vi "RobotRunTest 1 arm.vi"() -> ()   [LabVIEW 2016]
uses:
  EyeRobotDLL.dll
panel:
  in  "Auto Home":bool
  in  "KillControlProcess(for debug only)":bool
  out "ROBOT_KINEMATICS_NO_SOLUTION":bool
  out "ROBOT_KINEMATICS_INSERTION_LENGTH_TOO_SMALL":bool
  out "ROBOT_COMMAND_BEYONG_JOINT_RANGE":bool
  out "ROBOT_COMMAND_TOO_LARGE":bool
  out "ROBOT_COMMUNICATION_ERROR":bool
  out "ROBOT_NOT_RUNNING":bool
  out "ROBOT_HARDWARE_SENSOR_FAULT":bool
  out "ROBOT_HARDWARE_NOT_FOUND_ALL_DRIVES":bool
  out "ROBOT_HARDWARE_NOT_PRESENT":bool
  in  "ToolInsertionOffset":dbl=-54.76
  out "Homing XYZ Stage Done":bool
  out "Homing Tool Done":bool
  out "Homing Arm Done":bool
  out "Actual Tool Insertion Length":dbl
  in  "Tool Withdraw":bool
  in  "Target Tool Withdraw Speed":dbl=0.5
  in  "Target Tool Withdraw Length":dbl=-5.0
  in  "Set Tool Type":bool
  in  "ToolType":i32=6
  in  "Tool Fast Retraction":bool
  in  "Tool Insertion":bool
  in  "Target Tool Insertion Speed":dbl=0.5
  in  "Target Tool Insertion Length":dbl=10.0
  in  "Homing XYZ Stage":bool
  in  "Homing Tool":bool
  in  "Homing Arm":bool
  in  "XYZ Control or Joint Control":bool
  in  "E-STOP button":bool caption="Stop Button"
  in  "Robot Command":T1={"x"=0.0, "y"=0.0, "z"=-10.0, "roll"=0.0, "grasp"=0.0}
  in  "joint command":T2
  in  "Stop Labview Button":bool caption="Stop Button"
  in  "Run Pause":bool
  in  "XYZ Stage Power":bool
  in  "ArmPower":bool
  in  "XYZ Stage Command":cluster{"x":dbl, "y":dbl, "z":dbl}
  out "XYZ Stage Data":cluster{"x":dbl, "y":dbl, "z":dbl}
  out "Robot Data":T1
  out "ActualJointAngles (8 DOF)":T2
  out "RobotConnection Status":bool
  out "ReceiveCount":u64
  out "SendCount":u64
  # "Robot XYZ Command (kinematics included)"
  # "Joint Angle Command (for debug and testing)"
  # "Robot Status"
  # "XYZ Stage Position"
  # "Tool Insertion Commands"
  # "Homing Commands"
  # "Robot Errors"
  # "Tool Configuration Commands"
  # "For debug only, No need to use this button during labview operation, if does, then the low level control will be terminated, and everything will have to be rerestarted including homing"
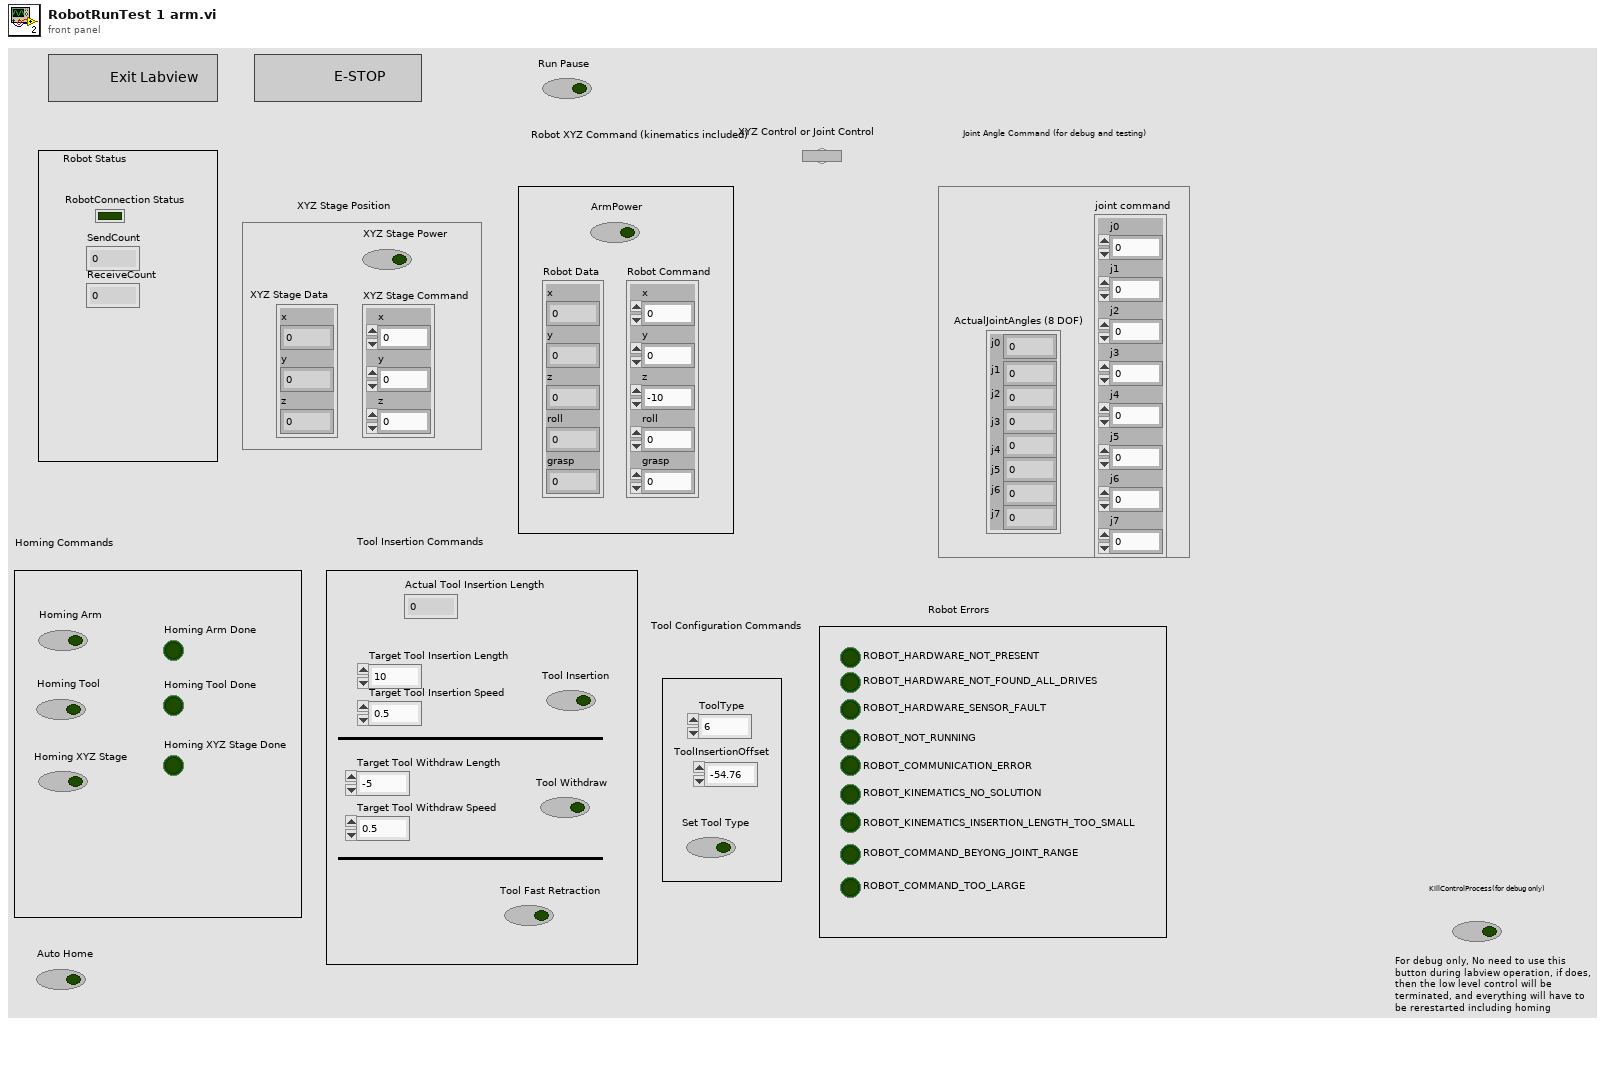
[diagram p1: front panel]
types:
  T1 = cluster{"x":dbl, "y":dbl, "z":dbl, "roll":dbl, "grasp":dbl}
  T2 = cluster{"j0":dbl, "j1":dbl, "j2":dbl, "j3":dbl, "j4":dbl, "j5":dbl, "j6":dbl, "j7":dbl}
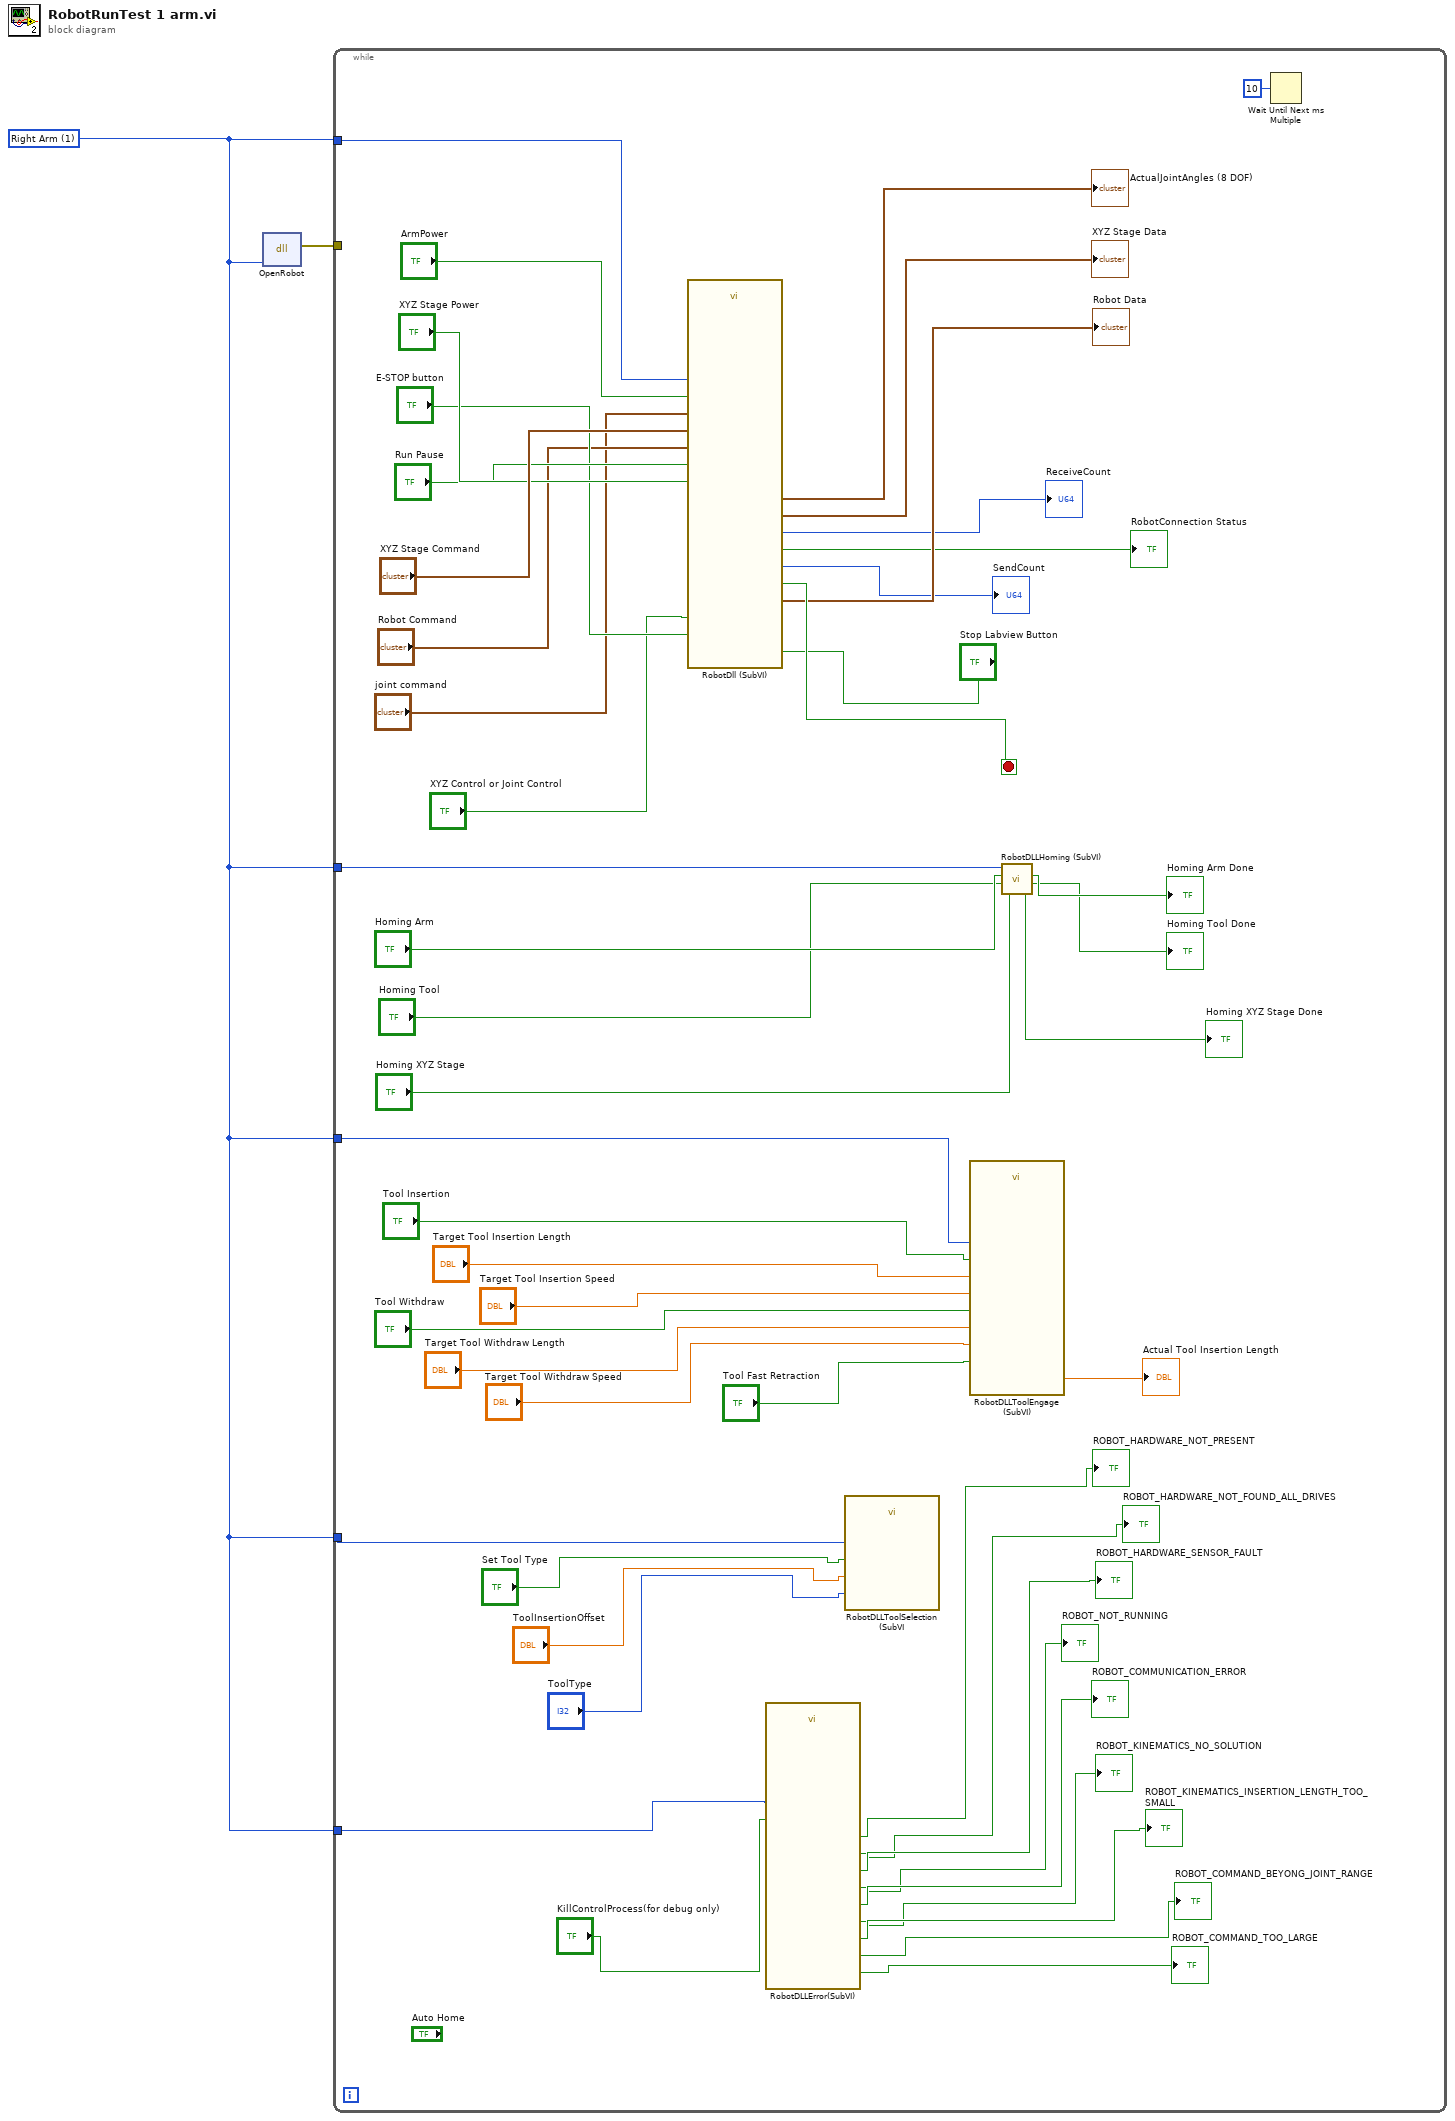
[diagram p0: block diagram]
diagram:
  w1 = u16 1 items=["Left Arm", "Right Arm"] ("Left or Right Arm")
  n1 = dll-call lib="D:/IRISS V2 dev/Host Demo/Functions/EyeRobotDLL.dll" fn="OpenRobot" label="Open"("id"=w1) -> (error out=w2:errorcluster)  [unwired: 5 in, 1 out]
  n2 = while {
    tunnel: w2 -> [_]
    tunnel: w1 -> [w45]
    tunnel: w1 -> [w24]
    tunnel: w1 -> [w33]
    tunnel: w1 -> [w7]
    tunnel: w1 -> [w3]
    stop <- w46 stop-if-true
    n3 = call "RobotDll (SubVI).vi"("rcm xyz command"="XYZ Stage Command", "ArmPower"="ArmPower", "Control Mode"="XYZ Control or Joint Control", "XYZ Stage Power"="XYZ Stage Power", "E-STOP button"="E-STOP button", "robot xyz command"="Robot Command", "ArmID"=w45, "Run"="Run Pause", "Stop Button in"="Stop Labview Button", "joint command"="joint command") -> ("rcm"=→"XYZ Stage Data":cluster{"x":dbl, "y":dbl, "z":dbl}, "Stop Button out"=w46:bool, "Tooltip"=→"Robot Data":T1, "ReceiveCount"=→"ReceiveCount":u64, "ActualJointAngles"=→"ActualJointAngles (8 DOF)":T2, "SendCount"=→"SendCount":u64, "RobotConnection"=→"RobotConnection Status":bool)  [unwired: 3 in]
    n4 = call "RobotDLLError(SubVI).vi"("ArmID"=w3, "KillRobotControlProcess"="KillControlProcess(for debug only)") -> ("ROBOT_COMMAND_BEYONG_JOINT_RANGE"=→"ROBOT_COMMAND_BEYONG_JOINT_RANGE":bool, "ROBOT_KINEMATICS_NO_SOLUTION"=→"ROBOT_KINEMATICS_NO_SOLUTION":bool, "ROBOT_HARDWARE_NOT_PRESENT"=→"ROBOT_HARDWARE_NOT_PRESENT":bool, "ROBOT_HARDWARE_NOT_FOUND_ALL_DRIVES"=→"ROBOT_HARDWARE_NOT_FOUND_ALL_DRIVES":bool, "ROBOT_HARDWARE_SENSOR_FAULT"=→"ROBOT_HARDWARE_SENSOR_FAULT":bool, "ROBOT_NOT_RUNNING"=→"ROBOT_NOT_RUNNING":bool, "ROBOT_COMMAND_TOO_LARGE"=→"ROBOT_COMMAND_TOO_LARGE":bool, "ROBOT_KINEMATICS_INSERTION_LENGTH_TOO_SMALL"=→"ROBOT_KINEMATICS_INSERTION_LENGTH_TOO_SMALL":bool, "ROBOT_COMMUNICATION_ERROR"=→"ROBOT_COMMUNICATION_ERROR":bool)  [unwired: 4 in, 1 out]
    n5 = call "RobotDLLToolSelection (SubVI.vi"("tool insertion offset"="ToolInsertionOffset", "ToolType"="ToolType", "Set Tool Type"="Set Tool Type", "ArmID"=w7) -> ()  [unwired: 4 in]
    n6 = call "RobotDLLToolEngage (SubVI).vi"("Tool Insertion"="Tool Insertion", "Tool Fast Retraction"="Tool Fast Retraction", "Target Tool Insertion Length"="Target Tool Insertion Length", "ArmID"=w33, "Target Tool Insertion Speed"="Target Tool Insertion Speed", "Tool Withdraw"="Tool Withdraw", "Target Tool Withdraw Length"="Target Tool Withdraw Length", "Target Tool Withdraw Speed"="Target Tool Withdraw Speed") -> ("actInsertionLength"=→"Actual Tool Insertion Length":dbl)  [unwired: 11 in]
    n7 = call "RobotDLLHoming (SubVI).vi"("Homing XYZ Stage"="Homing XYZ Stage", "Homing Tool"="Homing Tool", "Homing Arm"="Homing Arm", "ArmID"=w24) -> ("Homing XYZ Stage Done"=→"Homing XYZ Stage Done":bool, "Homing Tool Done"=→"Homing Tool Done":bool, "Homing Arm Done"=→"Homing Arm Done":bool)  [unwired: 1 in]
    n8 = Wait Until Next ms Multiple(millisecond multiple=u32 10) -> ()  [unwired: 1 out]
  }
